vi "close.vi"(8 "error in":errorcluster, 11 "Daqmx Module runtime in":refnum<class "DAQmx Module Runtime.lvclass">) -> (0 "error out":errorcluster)   [LabVIEW 2015, in "DAQmx Module Runtime.lvclass"]
doc: "Provides an interface for terminating a module instance. While this interface performs no operations, a child should close and deallocate any open references or memory."
uses:
  DAQmx Module Runtime.lvclass
  DAQmx Module Runtime.lvclass/DAQmx Module Runtime.ctl
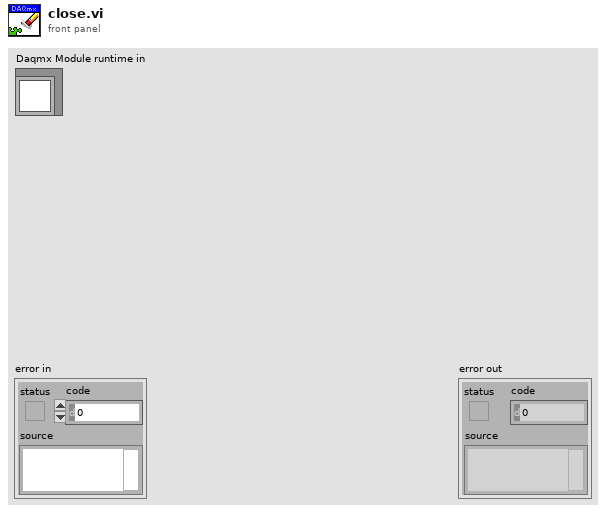
[diagram p1: front panel]
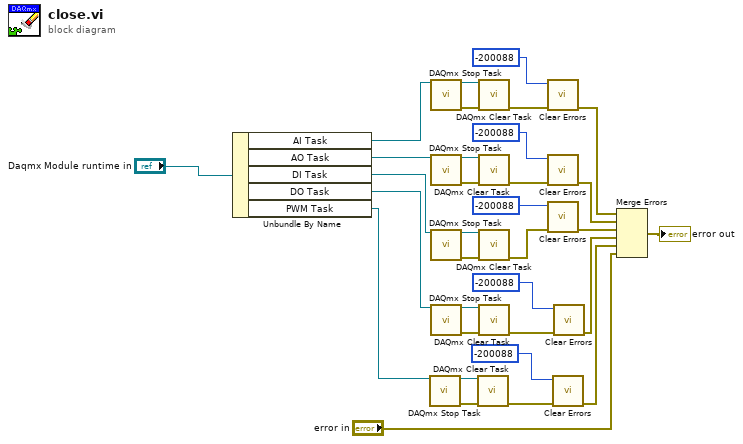
[diagram p0: block diagram]
diagram:
  n1 = Unbundle By Name("Daqmx Module runtime in") -> ("AI Task"=w27:refnum<k21>, "AO Task"=w26:refnum<k21>, "DI Task"=w25:refnum<k21>, "DO Task"=w24:refnum<k21>, "PWM Task"=w1:refnum<k21>)
  n2 = call <vilib>:"DAQmx Stop Task.vi"("task/channels in"=w1) -> ("task out"=w6:refnum<k21>, "error out"=w7:errorcluster)  [unwired: 13 in]
  n3 = call <vilib>:"DAQmx Stop Task.vi"("task/channels in"=w27) -> ("task out"=w23:refnum<k21>, "error out"=w33:errorcluster)  [unwired: 13 in]
  n4 = call <vilib>:"DAQmx Stop Task.vi"("task/channels in"=w26) -> ("task out"=w22:refnum<k21>, "error out"=w29:errorcluster)  [unwired: 13 in]
  n5 = call <vilib>:"DAQmx Stop Task.vi"("task/channels in"=w25) -> ("task out"=w21:refnum<k21>, "error out"=w30:errorcluster)  [unwired: 13 in]
  n6 = call <vilib>:"DAQmx Stop Task.vi"("task/channels in"=w24) -> ("task out"=w20:refnum<k21>, "error out"=w31:errorcluster)  [unwired: 13 in]
  n7 = call <vilib>:"DAQmx Clear Task.vi"("task in"=w6, "error in"=w7) -> ("error out"=w4:errorcluster)  [unwired: 13 in]
  n8 = call <vilib>:"DAQmx Clear Task.vi"("task in"=w23, "error in"=w33) -> ("error out"=w15:errorcluster)  [unwired: 13 in]
  n9 = call <vilib>:"DAQmx Clear Task.vi"("task in"=w22, "error in"=w29) -> ("error out"=w13:errorcluster)  [unwired: 13 in]
  n10 = call <vilib>:"DAQmx Clear Task.vi"("task in"=w21, "error in"=w30) -> ("error out"=w11:errorcluster)  [unwired: 13 in]
  n11 = call <vilib>:"DAQmx Clear Task.vi"("task in"=w20, "error in"=w31) -> ("error out"=w9:errorcluster)  [unwired: 13 in]
  n12 = call <vilib>:"Clear Errors.vi"("error in (no error)"=w15, "specific error code to clear (0: all)"=-200088) -> ("error out"=w14:errorcluster)  [unwired: 4 in, 1 out]
  n13 = call <vilib>:"Clear Errors.vi"("error in (no error)"=w13, "specific error code to clear (0: all)"=-200088) -> ("error out"=w12:errorcluster)  [unwired: 4 in, 1 out]
  n14 = call <vilib>:"Clear Errors.vi"("error in (no error)"=w11, "specific error code to clear (0: all)"=-200088) -> ("error out"=w10:errorcluster)  [unwired: 4 in, 1 out]
  n15 = call <vilib>:"Clear Errors.vi"("error in (no error)"=w4, "specific error code to clear (0: all)"=-200088) -> ("error out"=w3:errorcluster)  [unwired: 4 in, 1 out]
  n16 = call <vilib>:"Clear Errors.vi"("error in (no error)"=w9, "specific error code to clear (0: all)"=-200088) -> ("error out"=w8:errorcluster)  [unwired: 4 in, 1 out]
  n17 = Merge Errors(w14, w12, w10, w8, w3, "error in") -> (→"error out":errorcluster)
